vi "Write Analogue.vi"(8 "error in (no error)":errorcluster, 10 "Outbput":bool, 11 "PS in":refnum<class "APS7050.lvclass">) -> (0 "error out":errorcluster, 3 "PS out":refnum<class "APS7050.lvclass">)   [LabVIEW 2021, in "Concrete.lvlib" / "APS7050.lvclass"]
uses:
  APS7050.lvclass
  APS7050.lvclass/APS7050.ctl
  Harware Abstraction/AnalogIO/AIO.lvclass
  <instrlib>/APS-7000 Series/APS-7000 Series.lvlib
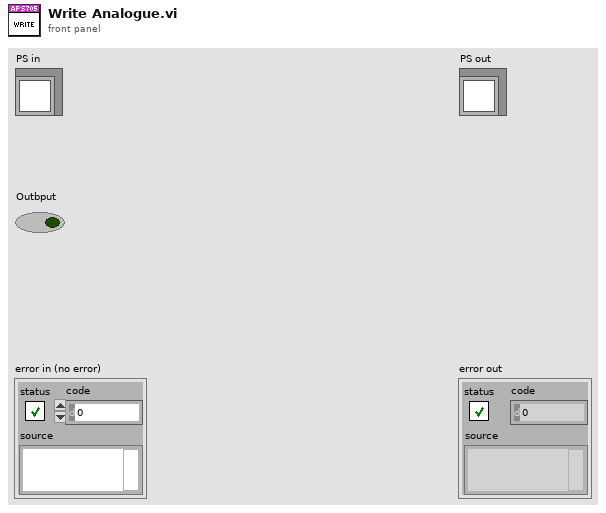
[diagram p1: front panel]
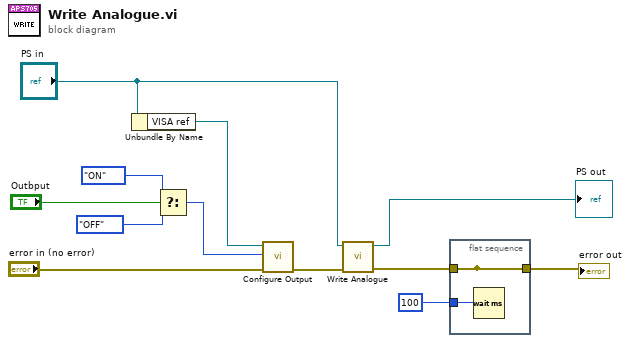
[diagram p0: block diagram]
diagram:
  n1 = Unbundle By Name("PS in") -> ("VISA ref"=w5:refnum<visa-resource-name>)
  n2 = Select(t=enum16{"OFF", "ON"}."ON" ("Output ON/OFF"), s="Outbput", f=enum16{"OFF", "ON"}."OFF" ("Output ON/OFF")) -> (s? t:f=w7:enum16{"OFF", "ON"})
  n3 = call <instrlib>:"Configure Output.vi"("error in"="error in (no error)", "Output ON/OFF"=w7, "VISA in"=w5) -> ("error out"=w4:errorcluster)  [unwired: 6 in, 2 out]
  n4 = call-parent "Write Analogue.vi"("error in (no error)"=w4, "PS in"="PS in") -> ("error out"=w2:errorcluster, "PS out"=→"PS out":refnum<class "APS7050.lvclass">)  [unwired: 8 in]
  n5 = flat-sequence {
    tunnel: [w13] -> _
    tunnel: w2 -> [w13]
    tunnel: u32 100 ("milliseconds to wait") -> [w14]
    tunnel: [w13] -> w1
    frame #0 {
      n6 = Wait (ms)(milliseconds to wait=w14) -> ()  [unwired: 1 out]
    }
  }
  "error out" <- w1
